vi "5.10 Manage Filter Threshold.vi"(1 "Output Control Signal":dbl, 2 "Gains and Parameters":T1, 3 "Filter Control":i32) -> (0 "Filter Value Output":dbl)   [LabVIEW 2010]
uses:
  5.10 Algorithm Parameters and Controls.ctl
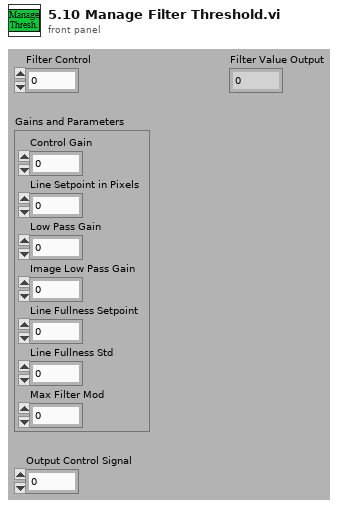
[diagram p1: front panel]
types:
  T1 = typedef "5.10 Algorithm Parameters and Controls.ctl" = cluster{"Control Gain":dbl, "Line Setpoint in Pixels":dbl, "Low Pass Gain":dbl, "Image Low Pass Gain":dbl, "Line Fullness Setpoint":dbl, "Line Fullness Std":dbl, "Max Filter Mod":dbl}
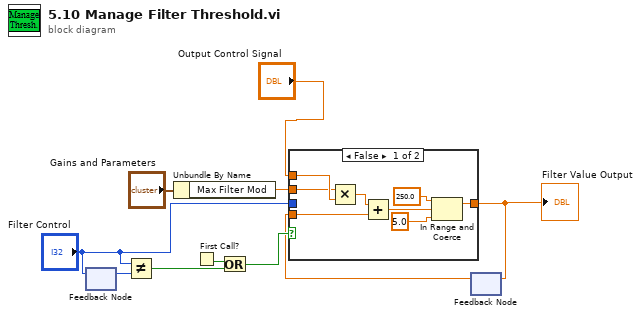
[diagram p0: block diagram]
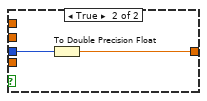
[diagram p2: hidden frame]
diagram:
  n1 = feedback #1() -> (w2:i32)  [unwired: 1 in]
  n2 = feedback-in #1("Filter Control") -> ()
  n3 = Not Equal?(x="Filter Control", y=w2) -> (x != y?=w3:bool)
  n4 = Unbundle By Name("Gains and Parameters") -> ("Max Filter Mod"=w10:dbl)
  n5 = First Call?() -> (First Call?: T/F=w8:bool)
  n6 = Or(x=w8, y=w3) -> (x .or. y?=w7:bool)
  n7 = feedback #2() -> (w6:dbl)  [unwired: 1 in]
  n8 = case shown="False" w7 {
    tunnel: [w15 w19] -> w5
    tunnel: "Filter Control" -> [_ w20]
    tunnel: w6 -> [w18 _]
    tunnel: "Output Control Signal" -> [w16 _]
    tunnel: w10 -> [w11 _]
    frame False {
      n9 = Multiply(x=w11, y=w16) -> (x*y=w12:dbl)
      n10 = Add(x=w12, y=w18) -> (x+y=w17:dbl)
      n11 = In Range and Coerce(upper limit=250.0, x=w17, lower limit=5.0) -> (coerced(x)=w15:dbl)  [unwired: 1 out]
    }
    frame True {
      n12 = To Double Precision Float(number=w20) -> (double precision float=w19:dbl)
    }
  }
  "Filter Value Output" <- w5
  n13 = feedback-in #2(w5) -> ()
